vi "Dashboard Cursor Interpolation.vi"(5 "Remove Cursor":bool, 7 "Add Cursor":bool, 9 "Graph Detail":i32, 10 "Interpolation Method":i32(ring)=1 items=["nearest", "linear", "spline", "cubic Hermite", "Lagrange"], 11 "Interpolation Points":refnum<vi>) -> ()   [LabVIEW 2018]
uses:
  <vilib>/Utility/miscctls.llb/LVCursorListTypeDef.ctl
  <vilib>/gmath/NI_Gmath.lvlib
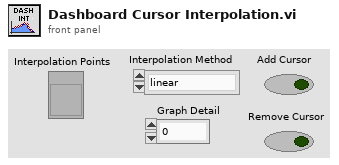
[diagram p1: front panel]
types:
  T1 = typedef "LVCursorListTypeDef.ctl" = cluster{"Name":string, "Color":u32, "Style":u8, "Point Style":u8, "Name Visible":bool, "Allow Drag":bool, "Cursor Mode":u32, "Plot":i32, "Index":i32, "Position":cluster{"X":dbl, "Y":dbl}, "X Scale":u32, "Y Scale":u32, "Watch Plots":i32[], "Watch All Plots":bool, "Plot Area":i32, "Label Offset":cluster{"X":dbl, "Y":dbl}}[]
  T2 = cluster{"Name":string, "Color":u32, "Style":u8, "Point Style":u8, "Name Visible":bool, "Allow Drag":bool, "Cursor Mode":u32, "Plot":i32, "Index":i32, "Position":cluster{"X":dbl, "Y":dbl}, "X Scale":u32, "Y Scale":u32, "Watch Plots":i32[], "Watch All Plots":bool, "Plot Area":i32, "Label Offset":cluster{"X":dbl, "Y":dbl}}
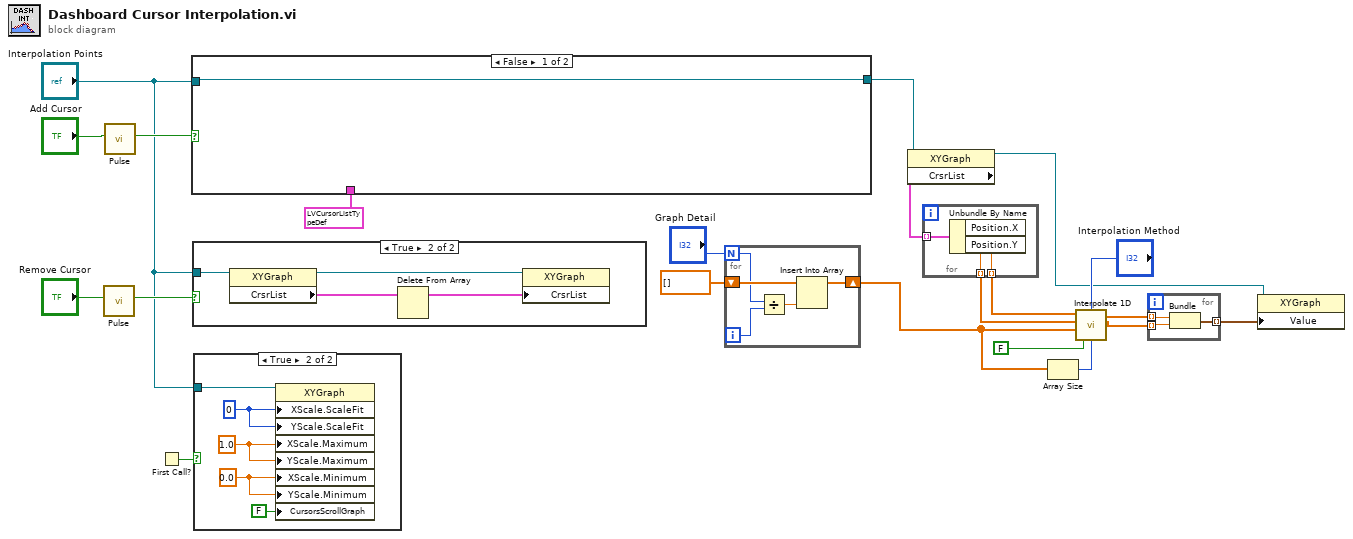
[diagram p0: block diagram]
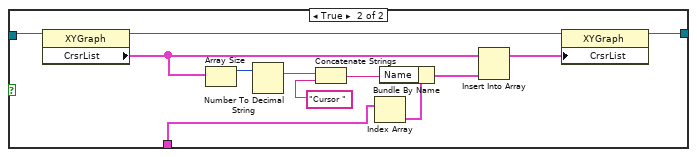
[diagram p4: hidden frame]
diagram:
  n1 = call "Pulse.vi"("Input"="Remove Cursor") -> ("Output"=w5:bool)  [unwired: 10 in]
  n2 = call "Pulse.vi"("Input"="Add Cursor") -> ("Output"=w3:bool)  [unwired: 10 in]
  n3 = First Call?() -> (First Call?: T/F=w2:bool)
  n4 = case shown="False" w3 {
    tunnel: T1 [{"Name"="Cursor 0", "Color"=33023, "Style"=0, "Point Style"=1, "Name Visible"=FALSE, "Allow Drag"=TRUE, "Cursor Mode"=0, "Plot"=0, "Index"=0, "Position"={"X"=0.5, "Y"=0.5}, "X Scale"=0, "Y Scale"=0, "Watch Plots"=[], "Watch All Plots"=FALSE, "Plot Area"=0, "Label Offset"={"X"=0.0, "Y"=0.0}}] ("Cursor List") -> [_ w31]
    tunnel: "Interpolation Points" -> [w22 w26]
    tunnel: [w22 w23] -> w8
    frame False {
    }
    frame True {
      n5 = property class="XYGraph"(reference=w26) -> (reference out=w25:refnum<vi>, "CrsrList"=w27:T1)  [unwired: 1 in, 1 out]
      n6 = Array Size(array=w27) -> (size(s)=w33:i32)
      n7 = Number To Decimal String(number=w33) -> (decimal integer string=w32:string)  [unwired: 1 in]
      n8 = Concatenate Strings("Cursor ", w32) -> (w29:string)
      n9 = Index Array(array=w31) -> (element=w30:T2)  [unwired: 1 in]
      n10 = Bundle By Name(cluster=w30, "Name"=w29) -> (w28:T2)
      n11 = Insert Into Array(array=w27, new element=w28) -> (w24:T1)  [unwired: 1 in]
      n12 = property class="XYGraph"(reference=w25, "CrsrList"=w24) -> (reference out=w23:refnum<vi>)  [unwired: 1 in, 1 out]
    }
  }
  n13 = case shown="True" w5 {
    tunnel: "Interpolation Points" -> [_ w36]
    frame False {
    }
    frame True {
      n14 = property class="XYGraph"(reference=w36) -> (reference out=w35:refnum<vi>, "CrsrList"=w37:T1)  [unwired: 1 in, 1 out]
      n15 = Delete From Array(array=w37) -> (array with subset deleted=w38:T1)  [unwired: 2 in, 1 out]
      n16 = property class="XYGraph"(reference=w35, "CrsrList"=w38) -> ()  [unwired: 1 in, 2 out]
    }
  }
  n17 = case shown="True" w2 {
    tunnel: "Interpolation Points" -> [_ w43]
    frame False {
    }
    frame True {
      w40 = 0.0 ("X Scale.Range:Maximum")
      w41 = 1.0 ("X Scale.Range:Maximum")
      w42 = u8 0 ("X Scale.Scale Fit")
      n18 = property class="XYGraph"(reference=w43, "XScale.ScaleFit"=w42, "YScale.ScaleFit"=w42, "XScale.Maximum"=w41, "YScale.Maximum"=w41, "XScale.Minimum"=w40, "YScale.Minimum"=w40, "CursorsScrollGraph"=FALSE ("Cursors Scroll Graph")) -> ()  [unwired: 1 in, 2 out]
    }
  }
  n19 = for {
    N: "Graph Detail" -> [w45]
    shift-right: [w47] -> w7
    shift-left: dbl[] [] -> [w46]
    i -> [w44]
    n20 = Divide(x=w44, y=w45) -> (x/y=w48:dbl)
    n21 = Insert Into Array(array=w46, new element=w48) -> (w47:dbl[])  [unwired: 1 in]
  }
  n22 = property class="XYGraph"(reference=w8) -> (reference out=w9:refnum<vi>, "CrsrList"=w13:T1)  [unwired: 1 in, 1 out]
  n23 = for {
    tunnel: w13 -> [w51] mode=indexing
    tunnel: [w50] -> w17 mode=indexing
    tunnel: [w49] -> w16 mode=indexing
    n24 = Unbundle By Name(w51) -> ("Position.X"=w50:dbl, "Position.Y"=w49:dbl)
  }
  n25 = Array Size(array=w7) -> (size(s)=w14:i32)
  n26 = call <vilib>:"Interpolate 1D.vi"("ntimes"=w14, "method"="Interpolation Method", "X is monotonic"=FALSE, "xi"=w7, "X"=w17, "Y"=w16) -> ("xi used"=w11:dbl[], "yi"=w12:dbl[])  [unwired: 3 in, 1 out]
  n27 = for {
    tunnel: w12 -> [w53] mode=indexing
    tunnel: w11 -> [w52] mode=indexing
    tunnel: [w54] -> w10 mode=indexing
    n28 = Bundle("Numeric"=w52, "Numeric"=w53) -> (w54:cluster{"Numeric":dbl, "Numeric":dbl})  [unwired: 1 in]
  }
  n29 = property class="XYGraph"(reference=w9, "Value"=w10) -> ()  [unwired: 1 in, 2 out]
